vi "csm_lumikki_instron_statusQue.vi"() -> ()   [LabVIEW 2009]
uses:
  <vilib>/Platform/ax-events.llb/Wait types.ctl
  Documents and Settings/All Users/Documents/Instron/FastTrack3/Common/MultiAxis/Arbitrator Interface/MX Arbitrator Globals.vi
panel:
  out "Event Queue 2":i32 format="%.0x"
  in  "error in (no error)":errorcluster
  out "Event Queue":u32
  in  "ARBY32Lib._DArby32":refnum<k7>(container)
  out "error out":errorcluster
  in  "Axis Information":T1(array[cluster])
  in  "Axis Selector":i32[](array[numeric])
  out "Item Names":string[](array[string])
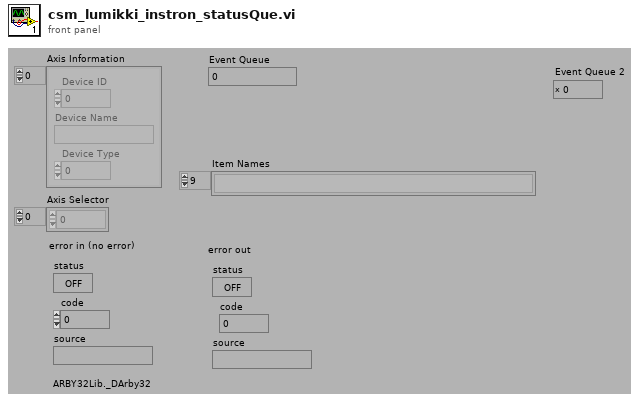
[diagram p1: front panel]
types:
  T1 = cluster{"Device ID":i32, "Device Name":string, "Device Type":i32}[]
  T2 = typedef "Wait types.ctl" = enum16{"Queued Mode", "Non Queued Mode"}
  T3 = cluster{"Axis Information[0]":cluster{"Device ID":i32, "Device Name":string, "Device Type":i32}, "Axis Information[1]":cluster{"Device ID":i32, "Device Name":string, "Device Type":i32}, "Axis Information[2]":cluster{"Device ID":i32, "Device Name":string, "Device Type":i32}, "Axis Information[3]":cluster{"Device ID":i32, "Device Name":string, "Device Type":i32}, "Axis Information[4]":cluster{"Device ID":i32, "Device Name":string, "Device Type":i32}, "Axis Information[5]":cluster{"Device ID":i32, "Device Name":string, "Device Type":i32}, "Axis Information[6]":cluster{"Device ID":i32, "Device Name":string, "Device Type":i32}, "Axis Information[7]":cluster{"Device ID":i32, "Device Name":string, "Device Type":i32}, "Axis Information[8]":cluster{"Device ID":i32, "Device Name":string, "Device Type":i32}}
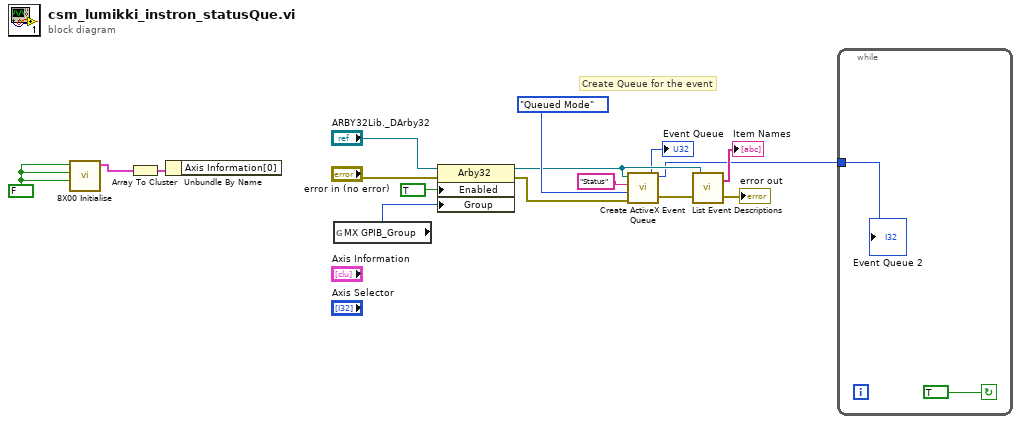
[diagram p0: block diagram]
diagram:
  w4 = FALSE ("Reset")
  # "Create Queue for the event"
  n1 = call "8X00 Initialise.vi"("Reset?"=w4, "Create DVM? (T)"=w4, "Create Console? (T)"=w4) -> ("Axis Information"=w3:T1)  [unwired: 1 in, 3 out]
  n2 = Array To Cluster(array=w3) -> (cluster=w2:T3)
  n3 = Unbundle By Name(w2) -> ()  [unwired: 1 out]
  n4 = global read "MX Arbitrator Globals.vi" "MX GPIB_Group"() -> (w15:i32)
  n5 = property class="Arby32"(reference="ARBY32Lib._DArby32", error in="error in (no error)", "Enabled"=TRUE, "Group"=w15) -> (reference out=w12:refnum<k7>, error out=w6:errorcluster)
  n6 = call <vilib>:"Create ActiveX Event Queue.vi"("error in (no error)"=w6, "Wait Options"=Wait_types."Queued Mode", "Event Name"="Status", "Automation Refnum"=w12) -> ("error out"=w8:errorcluster, "Event Queue"=w1:i32)  [unwired: 2 in]
  "Event Queue" <- w1
  n7 = call <vilib>:"List Event Descriptions.vi"("error in (no error)"=w8, "Automation Refnum"=w12) -> ("error out"=→"error out":errorcluster, "Function Descriptions"=→"Item Names":string[])
  n8 = while {
    tunnel: w1 -> [w17]
    stop <- TRUE continue-if-true
    "Event Queue 2" <- w17
  }
